vi "Initialize Generator.vi"(8 "error in":errorcluster, 11 "generator settings":T1={"Amplitude"=1.0, "Frequency"=10.0, "Sample Rate"=1000.0, "Noise Level"=0.0, "Signal Type"=enum."Sine", "Block Size"=100, "Update Interval ms"=100}) -> (0 "error out":errorcluster, 2 "generator settings out":T1={"Amplitude"=1.0, "Frequency"=10.0, "Sample Rate"=1000.0, "Noise Level"=0.0, "Signal Type"=enum."Sine", "Block Size"=100, "Update Interval ms"=100}, 3 "start sample":dbl)   [LabVIEW 2026, in "Signal Generator.lvlib"]
doc: "Initialization stage. Starts a new generation run: resets the absolute sample counter to zero so the first block begins at t = 0 with zero phase, and hands the validated generator settings on to the acquisition loop. The simulator uses no hardware, so there are no sessions or resources to open here."
uses:
  Signal Generator.lvlib
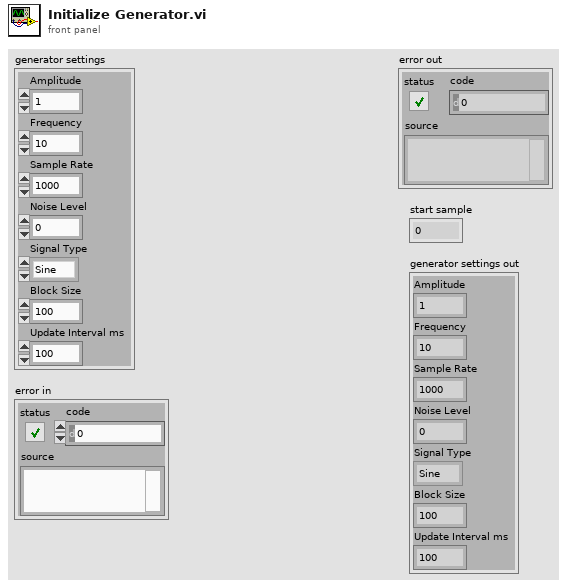
[diagram p1: front panel]
types:
  T1 = cluster{"Amplitude":dbl, "Frequency":dbl, "Sample Rate":dbl, "Noise Level":dbl, "Signal Type":enum32{"Sine", "Square", "Chirp"}, "Block Size":i32, "Update Interval ms":i32}
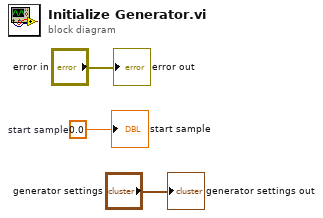
[diagram p0: block diagram]
diagram:
  w2 = 0.0  # start sample
  "error out" <- "error in"
  "start sample" <- w2
  "generator settings out" <- "generator settings"
